vi "GetVariableArray.vi"() -> (3 "Variable Array":T1(array[cluster]))   [LabVIEW 2012]
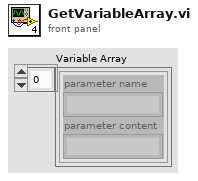
[diagram p1: front panel]
types:
  T1 = cluster{"parameter name":string, "parameter content":string}[]
  T2 = cluster{"parameter name":string, "parameter content":string}
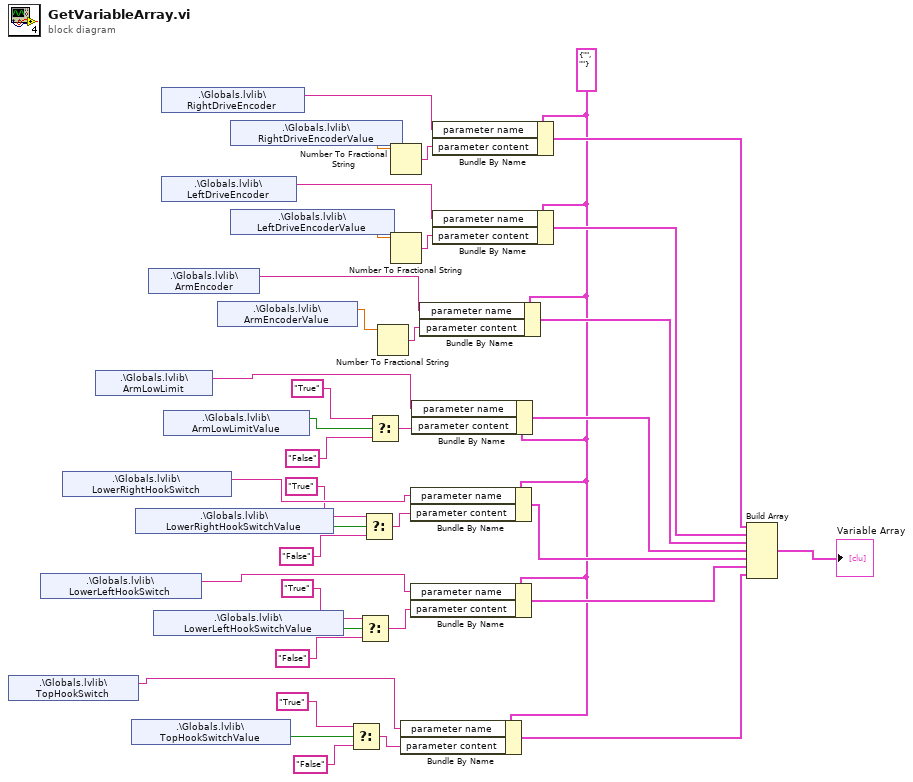
[diagram p0: block diagram]
diagram:
  w1 = T2 {"parameter name"="", "parameter content"=""}
  n1 = shared-variable ".\\Globals.lvlib\\TopHookSwitch"() -> (w33:string)  [unwired: 1 in, 1 out]
  n2 = shared-variable ".\\Globals.lvlib\\LowerLeftHookSwitch"() -> (w32:string)  [unwired: 1 in, 1 out]
  n3 = shared-variable ".\\Globals.lvlib\\LowerRightHookSwitch"() -> (w31:string)  [unwired: 1 in, 1 out]
  n4 = shared-variable ".\\Globals.lvlib\\ArmLowLimit"() -> (w26:string)  [unwired: 1 in, 1 out]
  n5 = shared-variable ".\\Globals.lvlib\\TopHookSwitchValue"() -> (w21:bool)  [unwired: 1 in, 1 out]
  n6 = shared-variable ".\\Globals.lvlib\\LowerRightHookSwitchValue"() -> (w16:bool)  [unwired: 1 in, 1 out]
  n7 = shared-variable ".\\Globals.lvlib\\ArmEncoder"() -> (w25:string)  [unwired: 1 in, 1 out]
  n8 = shared-variable ".\\Globals.lvlib\\LowerLeftHookSwitchValue"() -> (w18:bool)  [unwired: 1 in, 1 out]
  n9 = shared-variable ".\\Globals.lvlib\\RightDriveEncoder"() -> (w6:string)  [unwired: 1 in, 1 out]
  n10 = shared-variable ".\\Globals.lvlib\\LeftDriveEncoder"() -> (w7:string)  [unwired: 1 in, 1 out]
  n11 = shared-variable ".\\Globals.lvlib\\ArmLowLimitValue"() -> (w13:bool)  [unwired: 1 in, 1 out]
  n12 = shared-variable ".\\Globals.lvlib\\ArmEncoderValue"() -> (w24:dbl)  [unwired: 1 in, 1 out]
  n13 = shared-variable ".\\Globals.lvlib\\RightDriveEncoderValue"() -> (w5:dbl)  [unwired: 1 in, 1 out]
  n14 = shared-variable ".\\Globals.lvlib\\LeftDriveEncoderValue"() -> (w8:dbl)  [unwired: 1 in, 1 out]
  n15 = Select(t="True", s=w21, f="False") -> (s? t:f=w27:string)
  n16 = Select(t="True", s=w18, f="False") -> (s? t:f=w28:string)
  n17 = Select(t="True", s=w16, f="False") -> (s? t:f=w29:string)
  n18 = Select(t="True", s=w13, f="False") -> (s? t:f=w30:string)
  n19 = Number To Fractional String(number=w24) -> (F-format string=w10:string)  [unwired: 3 in]
  n20 = Number To Fractional String(number=w5) -> (F-format string=w4:string)  [unwired: 3 in]
  n21 = Number To Fractional String(number=w8) -> (F-format string=w9:string)  [unwired: 3 in]
  n22 = Bundle By Name(cluster=w1, "parameter name"=w33, "parameter content"=w27) -> (w38:T2)
  n23 = Bundle By Name(cluster=w1, "parameter name"=w31, "parameter content"=w29) -> (w36:T2)
  n24 = Bundle By Name(cluster=w1, "parameter name"=w32, "parameter content"=w28) -> (w37:T2)
  n25 = Bundle By Name(cluster=w1, "parameter name"=w26, "parameter content"=w30) -> (w35:T2)
  n26 = Bundle By Name(cluster=w1, "parameter name"=w25, "parameter content"=w10) -> (w34:T2)
  n27 = Bundle By Name(cluster=w1, "parameter name"=w6, "parameter content"=w4) -> (w2:T2)
  n28 = Bundle By Name(cluster=w1, "parameter name"=w7, "parameter content"=w9) -> (w3:T2)
  n29 = Build Array(w2, w3, w34, w35, w36, w37, w38) -> (→"Variable Array":T1)
